vi "getDisplacement.vi"(9 "Samples to Average":i32, 10 "Samples":i32, 11 "Sampling Frequency":dbl) -> (3 "max value":dbl)   [LabVIEW 2017]
panel:
  out "Numeric":i32
  out "XY Graph":cluster{"Y":dbl[], "Y":dbl[]}[](graph)
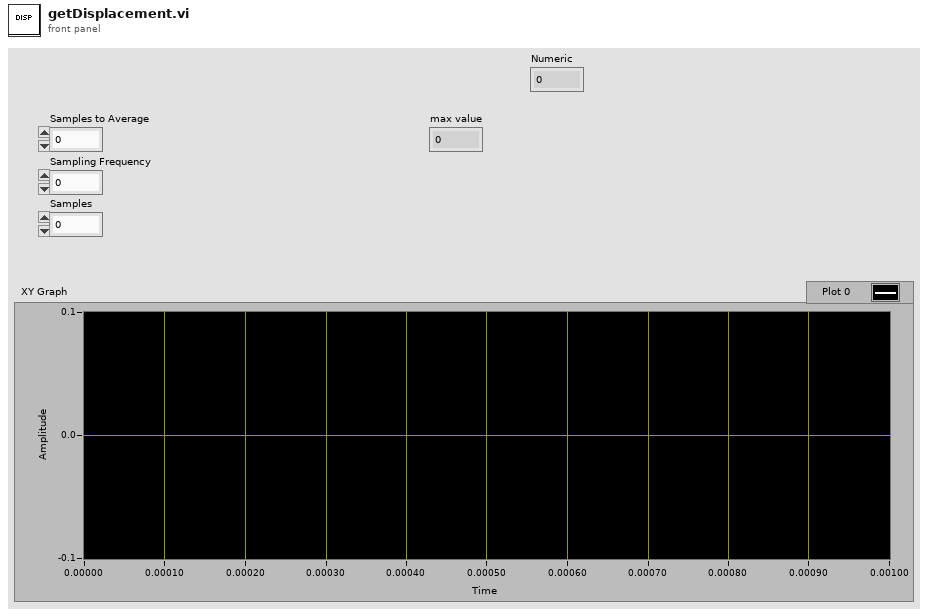
[diagram p1: front panel]
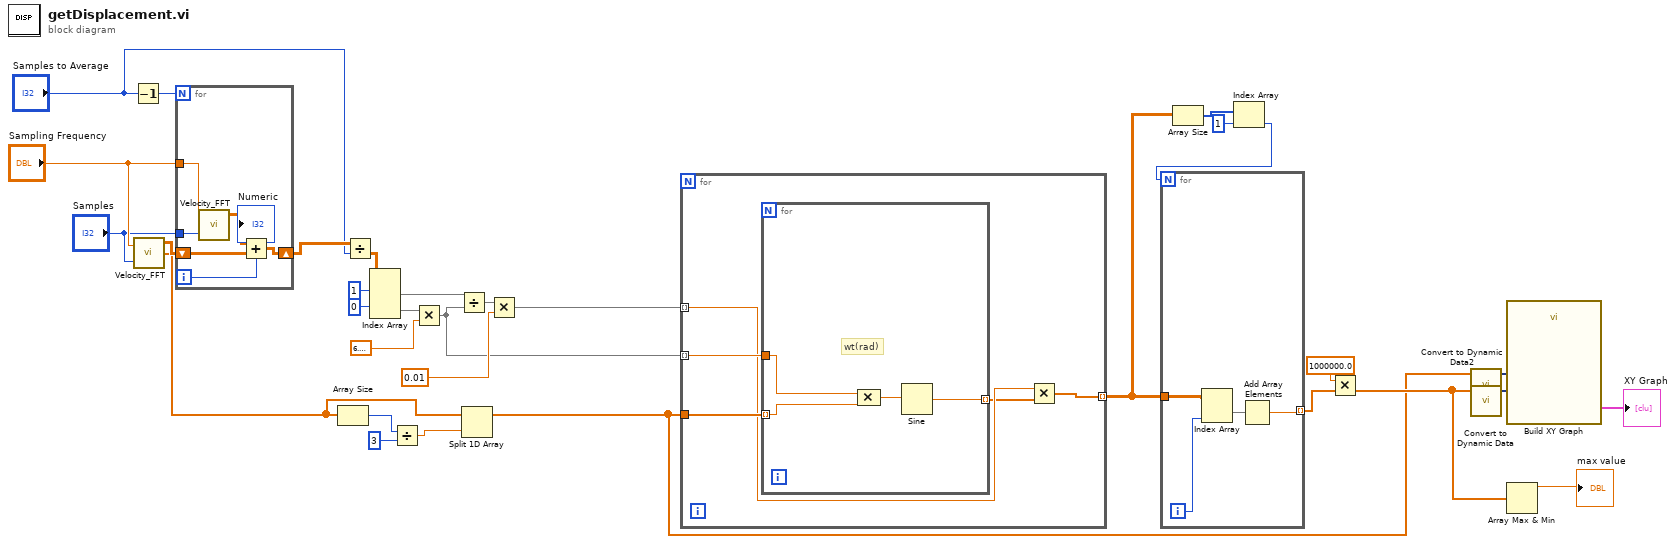
[diagram p0: block diagram]
diagram:
  n1 = Decrement(x="Samples to Average") -> (x-1=w28:i32)
  n2 = call "Velocity_FFT.vi"("Sampling Frequency"="Sampling Frequency", "Samples"="Samples") -> ("Peaks"=w21:dbl[][], "t_vect"=w6:dbl[])  [unwired: 1 out]
  n3 = for {
    N: w28 -> [_]
    tunnel: "Sampling Frequency" -> [w38]
    shift-right: [w36] -> w29
    shift-left: w21 -> [w37]
    tunnel: "Samples" -> [w35]
    i -> [w33]
    n4 = call "Velocity_FFT.vi"("Sampling Frequency"=w38, "Samples"=w35) -> ("Peaks"=w34:dbl[][])  [unwired: 2 out]
    n5 = Add(x=w34, y=w37) -> (x+y=w36:dbl[][])
    "Numeric" <- w33
  }
  n6 = Array Size(array=w6) -> (size(s)=w5:i32)
  n7 = Divide(x=w29, y="Samples to Average") -> (x/y=w30:dbl[][])
  n8 = Index Array(array=w30, index (row) #1=1 ("index (row)"), index (row) #2=0 ("index (row)")) -> (element #1=w22:dbl[], element #2=w20:dbl[])  [unwired: 2 in]
  n9 = Divide(x=w5, y=3) -> (x/y=w3:dbl)
  n10 = Multiply(x=w20, y=6.283185307179586) -> (x*y=w2:dbl[])
  n11 = Divide(x=w22, y=w2) -> (x/y=w24:dbl[])
  n12 = Split 1D Array(array=w6, index=w3) -> (first subarray=w7:dbl[])  [unwired: 1 out]
  n13 = Multiply(x=w24, y=0.01) -> (x*y=w19:dbl[])
  n14 = for {
    tunnel: w2 -> [w42] mode=indexing
    tunnel: w19 -> [w41] mode=indexing
    tunnel: w7 -> [w43]
    tunnel: [w40] -> w14 mode=indexing
    n15 = for {
      tunnel: w43 -> [w47] mode=indexing
      tunnel: w42 -> [w46]
      tunnel: [w44] -> w39 mode=indexing
      # "wt(rad)"
      n16 = Compound Arithmetic op=MULTIPLY(w46, w47) -> (w45:dbl)
      n17 = Sine(x=w45) -> (sin(x)=w44:dbl)
    }
    n18 = Multiply(x=w41, y=w39) -> (x*y=w40:dbl[])
  }
  n19 = Array Size(array=w14) -> (size(s)=w13:i32[])
  n20 = Index Array(array=w13, index=1) -> (element=w11:i32)
  n21 = for {
    N: w11 -> [_]
    tunnel: w14 -> [w51]
    tunnel: [w48] -> w17 mode=indexing
    i -> [w50]
    n22 = Index Array(array=w51, index (col)=w50) -> (element=w49:dbl[])  [unwired: 1 in]
    n23 = Add Array Elements(numeric array=w49) -> (sum=w48:dbl)
  }
  n24 = Multiply(x=1000000.0, y=w17) -> (x*y=w9:dbl[])
  n25 = call "Convert to Dynamic Data2"("Array"=w7) -> ("Dynamic Data Type"=w15:dynamicdata)  [unwired: 3 in]
  n26 = call "Convert to Dynamic Data"("Array"=w9) -> ("Dynamic Data Type"=w16:dynamicdata)  [unwired: 3 in]
  n27 = call "Build XY Graph"("Y Input"=w16, "X Input"=w15) -> ("XY Graph"=→"XY Graph":cluster{"X":dbl[], "Y":dbl[]}[])  [unwired: 8 in, 1 out]
  n28 = Array Max & Min(array=w9) -> (max value=→"max value":dbl)  [unwired: 3 out]
